vi "SubtractZeroes.vi"(10 "RawPressure":dbl[][](array[numeric]), 11 "Zeroes":dbl[](array[numeric])) -> (3 "ZeroedPressure":dbl[][](array[numeric]))   [LabVIEW 2013]
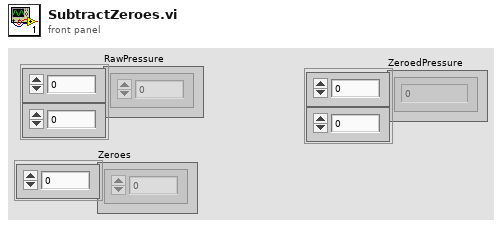
[diagram p1: front panel]
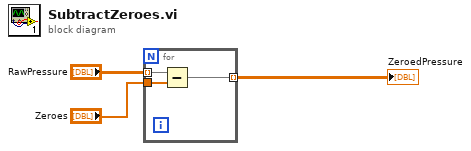
[diagram p0: block diagram]
diagram:
  n1 = for {
    tunnel: [w4] -> w1 mode=indexing
    tunnel: "RawPressure" -> [w6] mode=indexing
    tunnel: "Zeroes" -> [w5]
    n2 = Subtract(x=w6, y=w5) -> (x-y=w4:dbl[])
  }
  "ZeroedPressure" <- w1
